vi "2D Array to Excel 2012 NIVerified.vi"() -> ()   [LabVIEW 2016]
uses:
  <vilib>/Utility/NIReport.llb/Append Numeric Table to Report (wrap).vi
  <vilib>/Utility/NIReport.llb/NI_report.lvclass
  <vilib>/Utility/NIReport.llb/Excel/NI_Excel.lvclass
panel:
  out "error out":errorcluster
  in  "error in (no error)":errorcluster
  # "Overview: This example builds a 2D array of random numbers and writes this data to an Excel spreadsheet.\nRequirements:\nLabVIEW 2010 (or compatible)\nReport Generation Toolkit for Microsoft Office\nInstructions:\nRun this VI"
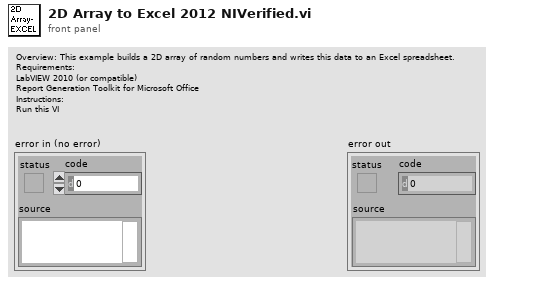
[diagram p1: front panel]
types:
  T1 = enum16{"Standard Report", "HTML", "Word", "Excel"}
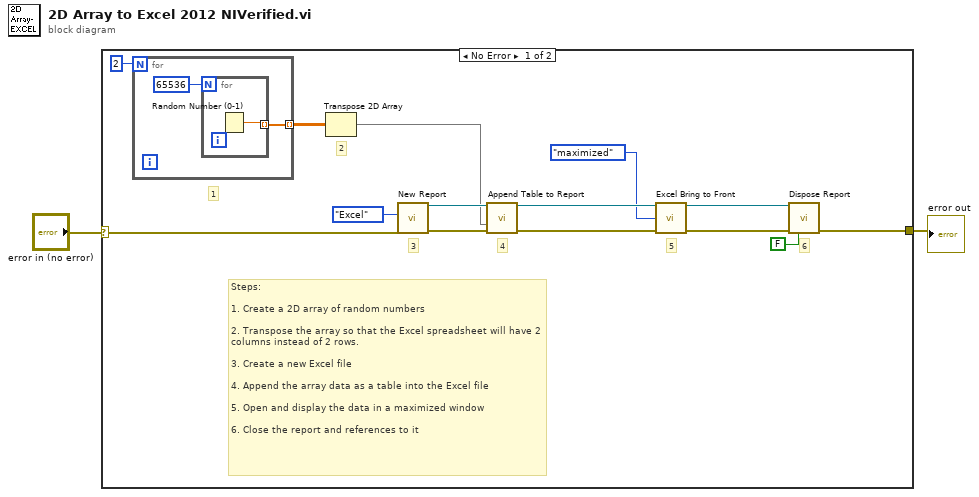
[diagram p0: block diagram]
diagram:
  n1 = case shown="No Error" "error in (no error)" {
    selector: "error in (no error)" -> [w3 w20]
    tunnel: [w4 w20] -> w2
    frame No Error {
      # "6"
      # "5"
      # "4"
      # "3"
      # "2"
      # "1"
      # "Steps:\n\n1. Create a 2D array of random numbers\n\n2. Transpose the array so that the Excel spreadsheet will have 2 \ncolumns instead of 2 rows.\n\n3. Create a new Excel file\n\n4. Append the array data as a table into the Excel file\n\n5. Open and display the data in a maximized window\n\n6. Close the report and references to it"
      n2 = for {
        N: 2 ("Numeric") -> [_]
        tunnel: [w18] -> w6 mode=indexing
        n3 = for {
          N: 65536 -> [_]
          tunnel: [w19] -> w18 mode=indexing
          n4 = Random Number (0-1)() -> (number: 0 to 1=w19:dbl)
        }
      }
      n5 = Transpose 2D Array(2D array=w6) -> (transposed array=w5:dbl[][])
      n6 = call <vilib>:"New Report.vi"("report type"=T1."Excel", "error in (no error)"=w3) -> ("report out"=w14:refnum<class "NI_report.lvclass">, "error out"=w13:errorcluster)  [unwired: 4 in, 8 out]
      n7 = call-poly <vilib>:"Append Table to Report.vi"("report in"=w14, "numerical data"=w5, "error in (no error)"=w13) -> ("report out"=w11:refnum<class "NI_report.lvclass">, "error out"=w10:errorcluster)  [unwired: 7 in, 4 out]
      n8 = call <vilib>:"Excel Bring to Front.vi"("report in"=w11, "window state (maximized)"=enum16{"maximized", "minimized", "normal"}."maximized", "error in (no error)"=w10) -> ("report out"=w8:refnum<class "NI_report.lvclass">, "error out"=w9:errorcluster)  [unwired: 11 out]
      n9 = call-dynamic "Dispose Report.vi"("report in"=w8, "error in (no error)"=w9, "close report? (T)"=FALSE) -> ("error out"=w4:errorcluster)  [unwired: 2 in, 10 out]
    }
    frame Error {
    }
  }
  "error out" <- w2
